vi "SearchAndReplaceCharacters.vi"(7 "CharactersToSearch":string, 10 "CharacterToReplace":string, 11 "StringIn":string) -> (3 "ResultString":string)   [LabVIEW 2021]
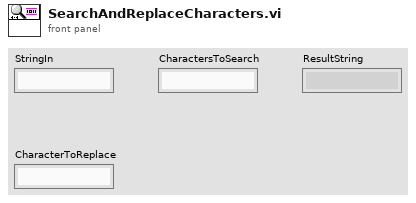
[diagram p1: front panel]
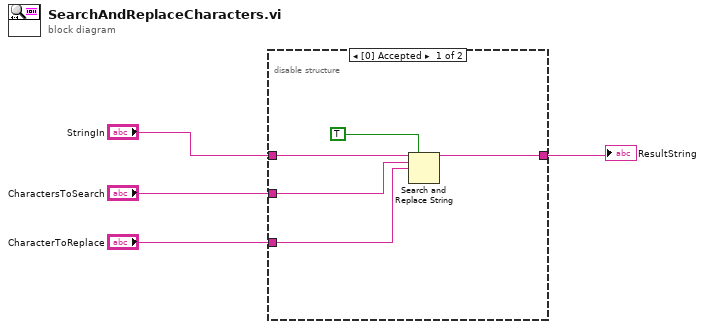
[diagram p0: block diagram]
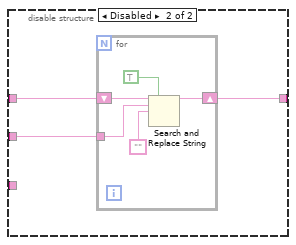
[diagram p2: hidden frame]
diagram:
  n1 = disable-structure shown="[0] Accepted" {
    disable-tunnel: "StringIn" -> [w9 w12]
    disable-tunnel: [w8 w11] -> w3
    disable-tunnel: "CharactersToSearch" -> [w6 w10]
    disable-tunnel: "CharacterToReplace" -> [w5 _]
    frame Enabled {
      n2 = Search and Replace String(replace all?=TRUE ("replace all? (F)"), input string=w9, search string=w6, replace string=w5) -> (result string=w8:string)  [unwired: 4 in, 3 out]
    }
    frame Disabled {
      n3 = for {
        tunnel: w10 -> [w14]
        shift-right: [w16] -> w11
        shift-left: w12 -> [w17]
        n4 = Search and Replace String(replace all?=TRUE ("replace all? (F)"), input string=w17, search string=w14, replace string="") -> (result string=w16:string)  [unwired: 4 in, 3 out]
      }
    }
  }
  "ResultString" <- w3
